vi "OpenTutorial_LandingPage.vi"   [LabVIEW 2021]
uses:
  <vilib>/Platform/browser.llb/Open URL in Default Browser (string).vi
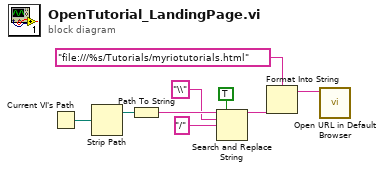
[diagram p0: block diagram]
diagram:
  n1 = Current VI's Path() -> (path=w2:path)
  n2 = Strip Path(path=w2) -> (stripped path=w3:path)  [unwired: 1 out]
  n3 = Path To String(path=w3) -> (string=w7:string)
  n4 = Search and Replace String(replace all?=TRUE ("replace all? (F)"), input string=w7, search string="\\", replace string="/" ("replace string (\"\")")) -> (result string=w6:string)  [unwired: 4 in, 3 out]
  n5 = Format Into String(format string="file:///%s/Tutorials/myriotutorials.html", w6) -> (resulting string=w8:string)  [unwired: 2 in, 1 out]
  n6 = call-poly <vilib>:"Open URL in Default Browser.vi"("URL"=w8) -> ()  [unwired: 5 in, 2 out]
